vi "SetExposureTime.vi"(9 "ExposureTime":refnum<k24>, 10 "Settings":refnum<k24>, 11 "Digital in":refnum<vi>) -> ()   [LabVIEW 2018]
uses:
  D:/SVN/PM/sdk/AppSamples/LabVIEWSamples/trunk/Release/2018/Dependencies/PVCamNET.dll
  Dependencies/PVCamNET.dll
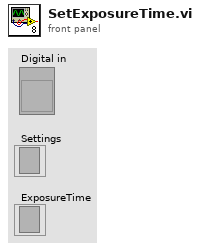
[diagram p1: front panel]
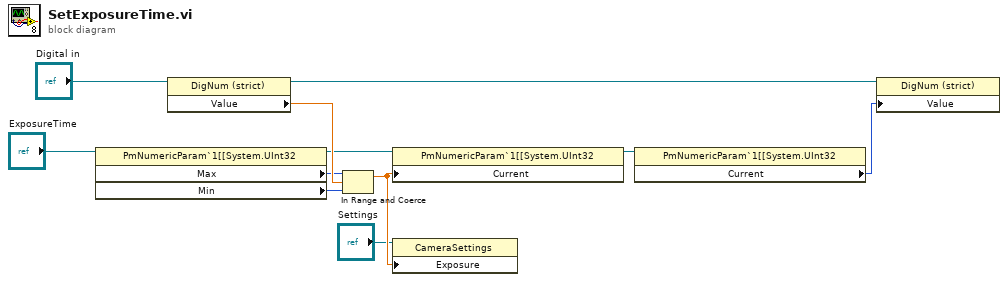
[diagram p0: block diagram]
diagram:
  n1 = property class="PmNumericParam`1[[System.UInt32"(reference="ExposureTime") -> (reference out=w4:refnum<k24>, "Max"=w2:u32, "Min"=w3:u32)  [unwired: 1 in, 1 out]
  n2 = property class="DigNum (strict)"(reference="Digital in") -> (reference out=w10:refnum<vi>, "Value"=w9:dbl)  [unwired: 1 in, 1 out]
  n3 = In Range and Coerce(upper limit=w2, x=w9, lower limit=w3) -> (coerced(x)=w7:dbl)  [unwired: 1 out]
  n4 = property class="PmNumericParam`1[[System.UInt32"(reference=w4, "Current"=w7) -> (reference out=w5:refnum<k24>)  [unwired: 1 in, 1 out]
  n5 = property class="CameraSettings"(reference="Settings", "Exposure"=w7) -> ()  [unwired: 1 in, 2 out]
  n6 = property class="PmNumericParam`1[[System.UInt32"(reference=w5) -> ("Current"=w11:u32)  [unwired: 1 in, 2 out]
  n7 = property class="DigNum (strict)"(reference=w10, "Value"=w11) -> ()  [unwired: 1 in, 2 out]
